vi "Read Thing Name.vi"(8 "error in (no error)":errorcluster, 11 "Shadow Thing in":refnum<class "Thing Shadow.lvclass">) -> (0 "error out":errorcluster, 2 "Thing Name":string, 3 "Shadow Thing out":refnum<class "Thing Shadow.lvclass">)   [LabVIEW 2015, in "NI_AWS_IoT.lvlib" / "Thing Shadow.lvclass"]
uses:
  Thing Shadow.lvclass
  Thing Shadow.lvclass/Thing Shadow.ctl
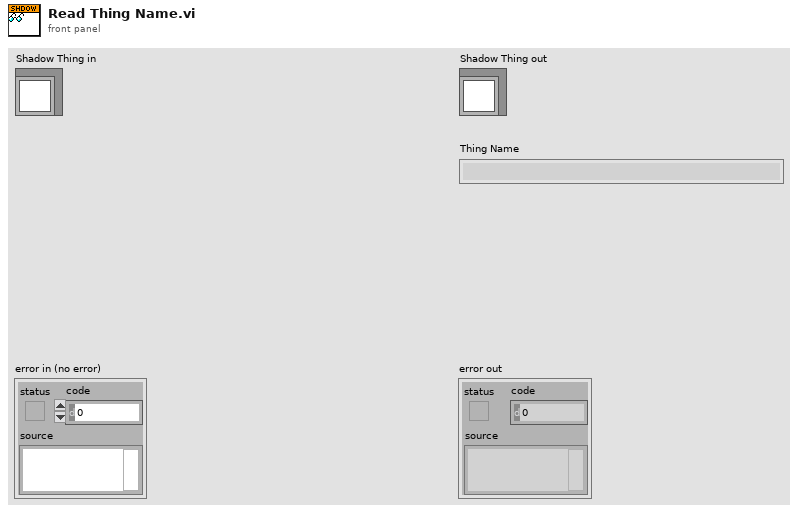
[diagram p1: front panel]
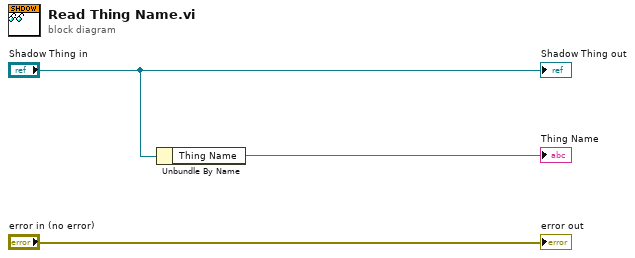
[diagram p0: block diagram]
diagram:
  n1 = Unbundle By Name("Shadow Thing in") -> ("Thing Name"=→"Thing Name":string)
  "error out" <- "error in (no error)"
  "Shadow Thing out" <- "Shadow Thing in"
